vi "FPGAUpdateAIO_DIO.vi"(1 "DIO cluster":T2, 2 "AIO cluster":T1) -> ()   [LabVIEW 2017]
panel:
  # "AOM"
  # "MW7"
  # "MW8"
  # "XM"
  # "XR"
  # "AOM"
  # "EOM"
  # "MW"
  # "MW1"
  # "MW2"
  # "MW3"
  # "MW4"
  # "MW5"
  # "MW6"
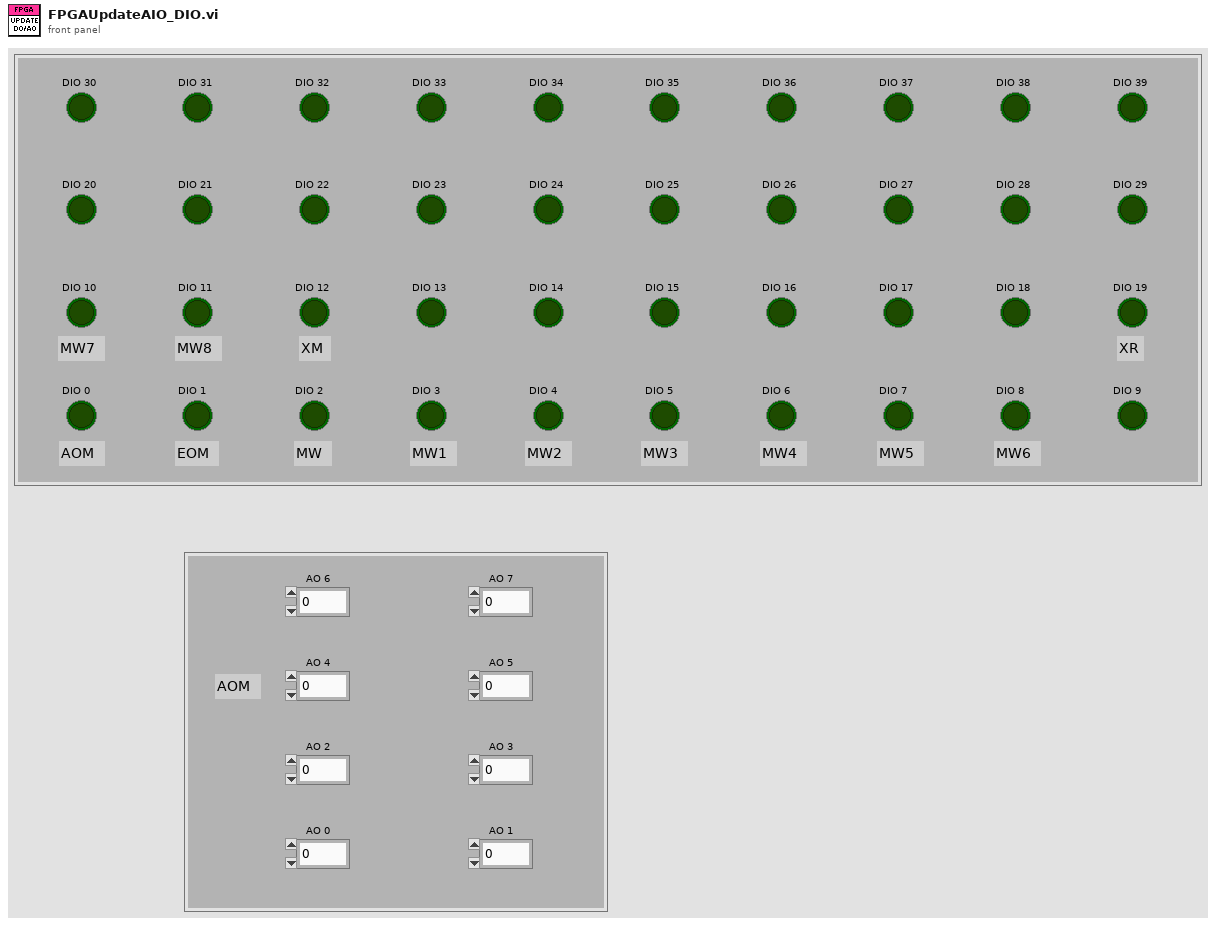
[diagram p1: front panel]
types:
  T1 = cluster{"AO 0":dbl, "AO 1":dbl, "AO 2":dbl, "AO 3":dbl, "AO 4":dbl, "AO 5":dbl, "AO 6":dbl, "AO 7":dbl}
  T2 = cluster{"DIO 30":bool, "DIO 31":bool, "DIO 32":bool, "DIO 33":bool, "DIO 34":bool, "DIO 35":bool, "DIO 36":bool, "DIO 37":bool, "DIO 38":bool, "DIO 39":bool, "DIO 20":bool, "DIO 21":bool, "DIO 22":bool, "DIO 23":bool, "DIO 24":bool, "DIO 25":bool, "DIO 26":bool, "DIO 27":bool, "DIO 28":bool, "DIO 29":bool, "DIO 10":bool, "DIO 11":bool, "DIO 12":bool, "DIO 13":bool, "DIO 14":bool, "DIO 15":bool, "DIO 16":bool, "DIO 17":bool, "DIO 18":bool, "DIO 19":bool, "DIO 0":bool, "DIO 1":bool, "DIO 2":bool, "DIO 3":bool, "DIO 4":bool, "DIO 5":bool, "DIO 6":bool, "DIO 7":bool, "DIO 8":bool, "DIO 9":bool}
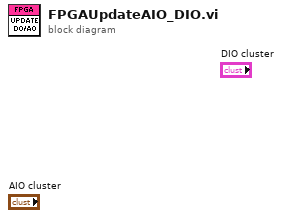
[diagram p0: block diagram]
diagram:
